vi "Pre-Build Custom Action.vi"(10 "Variant":variant) -> (0 "error out":errorcluster)   [LabVIEW 2019]
uses:
  <vilib>/Utility/traverseref.llb/TRef TravTarget.ctl
  src/Lockin.Utilities/Application Version.vi
  <vilib>/Utility/traverseref.llb/VI Scripting - Traverse.lvlib
  src/Lockin.Utilities/Lockin.Utilities.lvlib
  <vilib>/LabVIEW Open Source Project/Unicity/RandomStringGenerator/RandomStringGenerator.lvclass
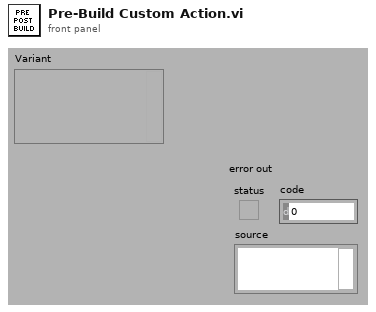
[diagram p1: front panel]
types:
  T1 = typedef "TRef TravTarget.ctl" = enum16{"FP", "BD", "Other"}
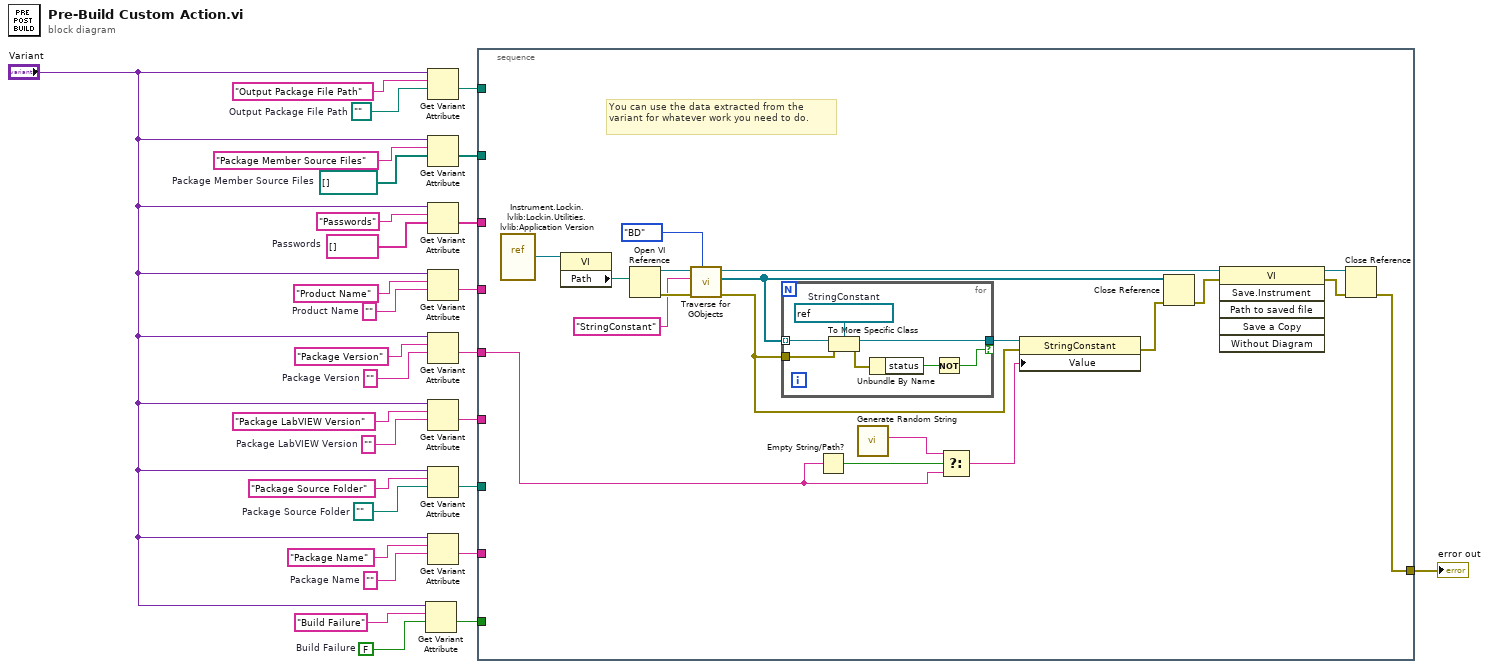
[diagram p0: block diagram]
diagram:
  w4 = FALSE  # Build Failure
  w14 = path ""  # Package Source Folder
  w15 = ""  # Package Name
  w18 = ""  # Package LabVIEW Version
  w20 = ""  # Package Version
  w22 = ""  # Product Name
  w24 = string[] []  # Passwords
  w26 = path[] []  # Package Member Source Files
  w28 = path ""  # Output Package File Path
  n1 = Get Variant Attribute(Variant="Variant", name="Build Failure", default value (empty Variant)=w4) -> (value=w2:bool)  [unwired: 1 in, 3 out]
  n2 = Get Variant Attribute(Variant="Variant", name="Output Package File Path", default value (empty Variant)=w28) -> (value=w13:path)  [unwired: 1 in, 3 out]
  n3 = Get Variant Attribute(Variant="Variant", name="Package Member Source Files", default value (empty Variant)=w26) -> (value=w12:path[])  [unwired: 1 in, 3 out]
  n4 = Get Variant Attribute(Variant="Variant", name="Passwords", default value (empty Variant)=w24) -> (value=w11:string[])  [unwired: 1 in, 3 out]
  n5 = Get Variant Attribute(Variant="Variant", name="Product Name", default value (empty Variant)=w22) -> (value=w10:string)  [unwired: 1 in, 3 out]
  n6 = Get Variant Attribute(Variant="Variant", name="Package Version", default value (empty Variant)=w20) -> (value=w9:string)  [unwired: 1 in, 3 out]
  n7 = Get Variant Attribute(Variant="Variant", name="Package LabVIEW Version", default value (empty Variant)=w18) -> (value=w8:string)  [unwired: 1 in, 3 out]
  n8 = Get Variant Attribute(Variant="Variant", name="Package Source Folder", default value (empty Variant)=w14) -> (value=w7:path)  [unwired: 1 in, 3 out]
  n9 = Get Variant Attribute(Variant="Variant", name="Package Name", default value (empty Variant)=w15) -> (value=w6:string)  [unwired: 1 in, 3 out]
  n10 = stacked-sequence {
    tunnel: w13 -> [_]
    tunnel: w12 -> [_]
    tunnel: w11 -> [_]
    tunnel: w10 -> [_]
    tunnel: w9 -> [w32]
    tunnel: w8 -> [_]
    tunnel: w7 -> [_]
    tunnel: w6 -> [_]
    tunnel: w2 -> [_]
    tunnel: [w34] -> w1
    frame #0 {
      # "You can use the data extracted from the variant for whatever work you need to do."
      n11 = vi-ref "Instrument.Lockin.lvlib:Lockin.Utilities.lvlib:Application Version.vi"() -> (w43:refnum<vi>)
      n12 = property class="VI"(reference=w43) -> ("Path"=w44:path)  [unwired: 1 in, 2 out]
      n13 = Open VI Reference(vi path=w44) -> (vi reference=w38:refnum<vi>, error out=w40:errorcluster)  [unwired: 5 in]
      n14 = call <vilib>:"Traverse for GObjects.vi"("Traverse Target"=TRef_TravTarget."BD", "error in (no error)"=w40, "Class Name"="StringConstant", "VI Refnum"=w38) -> ("error out"=w42:errorcluster, "References"=w41:refnum<vi>[], "dup VI Refnum"=w45:refnum<vi>)  [unwired: 4 in, 1 out]
      n15 = for {
        tunnel: w41 -> [w55] mode=indexing
        tunnel: [w54] -> w39 if=w51
        tunnel: w42 -> [w53]
        w50 = refnum<vi> refnum  # StringConstant
        n16 = To More Specific Class(target class=w50, reference=w55, error in=w53) -> (specific class reference=w54:refnum<vi>, error out=w49:errorcluster)
        n17 = Unbundle By Name(w49) -> ("status"=w52:bool)
        n18 = Not(x=w52) -> (.not. x?=w51:bool)
      }
      n19 = Empty String/Path?(string/path=w32) -> (empty?=w33:bool)
      n20 = call <vilib>:"Generate Random String.vi"() -> ("Random String"=w30:string)  [unwired: 11 in]
      n21 = Select(t=w30, s=w33, f=w32) -> (s? t:f=w31:string)
      n22 = property on="Property Node" class="StringConstant"(reference=w39, error in=w42, "Value"=w31) -> (error out=w37:errorcluster)  [unwired: 1 out]
      n23 = Close Reference(reference=w41, error in (no error)=w37) -> (error out=w47:errorcluster)
      n24 = invoke class="VI" method="Save.Instrument"(reference=w45, error in=w47) -> (reference out=w46:refnum<vi>, error out=w48:errorcluster)  [unwired: 4 in, 4 out]
      n25 = Close Reference(reference=w46, error in (no error)=w48) -> (error out=w34:errorcluster)
    }
  }
  "error out" <- w1
